vi "Write Instr.vi"(8 "error in (no error)":errorcluster, 10 "Instr":refnum<class "Instrument.lvclass">, 11 "Instrument Actor in":refnum<class "Instrument Actor.lvclass">) -> (0 "error out":errorcluster, 3 "Instrument Actor out":refnum<class "Instrument Actor.lvclass">)   [LabVIEW 2016, in "Instrument Actor.lvclass"]
uses:
  Instrument Actor.lvclass
  Instrument.lvclass
  Instrument Actor.lvclass/Instrument Actor.ctl
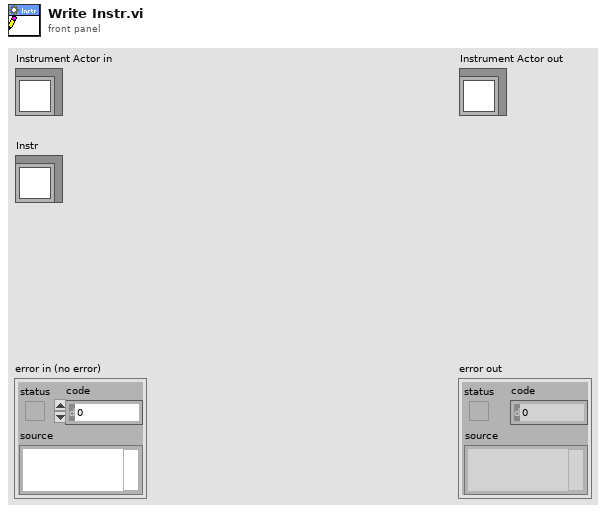
[diagram p1: front panel]
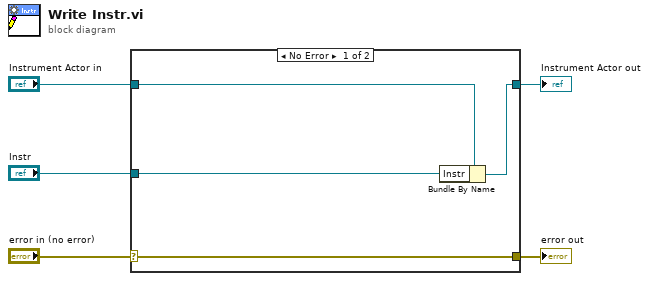
[diagram p0: block diagram]
diagram:
  n1 = case shown="No Error" "error in (no error)" {
    selector: "error in (no error)" -> [w9 w10]
    tunnel: [w9 w10] -> w4
    tunnel: [w7 w11] -> w2
    tunnel: "Instrument Actor in" -> [w8 w11]
    tunnel: "Instr" -> [w6 _]
    frame No Error {
      n2 = Bundle By Name(cluster=w8, "Instr"=w6) -> (w7:refnum<class "Instrument Actor.lvclass">)
    }
    frame Error {
    }
  }
  "error out" <- w4
  "Instrument Actor out" <- w2
